vi "Run Test.vi"(8 "error in (no error)":errorcluster, 11 "Test Template in":refnum<class "Instrument Setup.lvclass">) -> (0 "error out":errorcluster, 1 "Positions":i32[](array[numeric]), 2 "Tests Passed":bool[](array[boolean]), 3 "Test Template out":refnum<class "Instrument Setup.lvclass">, 5 "Fail Codes":string[](array[string]))   [LabVIEW 2015, in "Instrument Setup.lvclass"]
doc: "Setup Loads, DPMs, Power Supplies, and Switch."
uses:
  Instrument Setup.lvclass
  CBTF Applications/Driver Board Testing/Main/Application/Application/Class/typedefs/Instrument Selector -- Enum.ctl
  Test Class/Test Class.lvclass
  CBTF Applications/Driver Board Testing/Main/Application/Application/Class/Driver Board Test.lvclass
  Classes/Application/Class/Application.lvclass
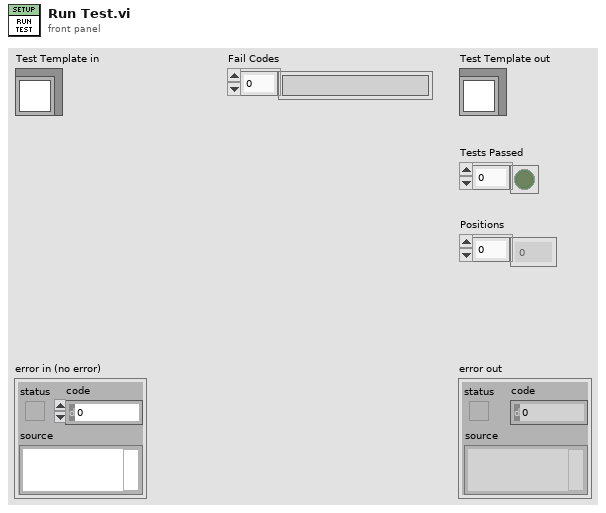
[diagram p1: front panel]
types:
  T1 = typedef "Driver Board Test.lvlib/Driver Board Test.lvclass/Instrument Selector -- Enum.ctl" = enum16{"ACPS1", "ACPS2", "DCPS1", "DCPS2", "DCPS3", "DCLoad1", "DCLoad2", "DPM1", "DPM2", "Switch1", "PXI1Slot2", "PXI1Slot3", "cDAQ1Mod5", "cDAQ1Mod6", "cDAQ1Mod7", "cDAQ1Mod8", "cDAQ1Mod1", "cDAQ1Mod2", "cDAQ1Mod3", "cDAQ1Mod4", "cDAQ2Mod1", "cDAQ2Mod2", "cDAQ2Mod3", "cDAQ2Mod4"}
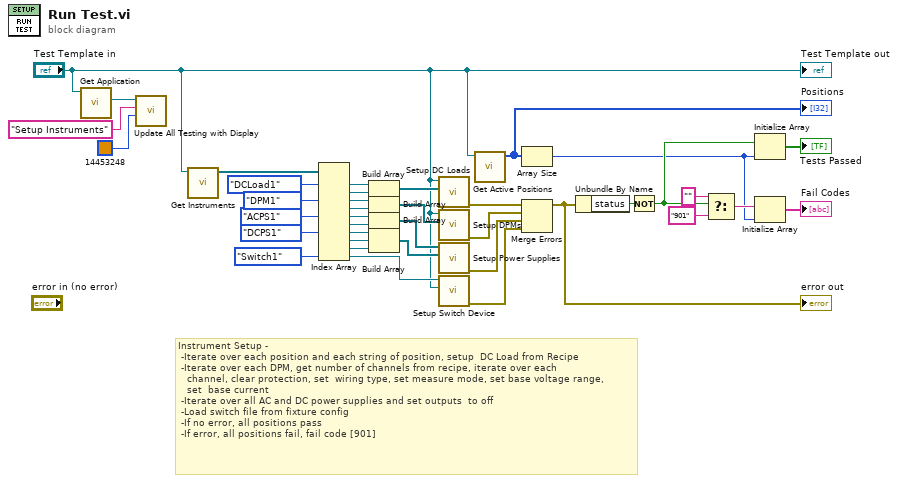
[diagram p0: block diagram]
diagram:
  # "Instrument Setup - \n\t-Iterate over each position and each string of position, setup \tDC Load from Recipe\n\t-Iterate over each DPM, get number of channels from\trecipe, iterate over each \n   channel, clear protection, set \twiring type, set measure mode, set base voltage range, \n   set \tbase current\n\t-Iterate over all AC and DC power supplies and set outputs \tto off\n\t-Load switch file from fixture config\n\t-If no error, all positions pass\n\t-If error, all positions fail, fail code [901]"
  n1 = call "Get Application.vi"("Test Class in"="Test Template in") -> ("Application.lvlib:Application.lvclass"=w7:refnum<class "Application.lvclass">)  [unwired: 9 in, 1 out]
  n2 = call "Update All Testing with Display.vi"("BG Color"=u32 14453248, "Message ('')"="Setup Instruments", "Application in"=w7) -> ()  [unwired: 7 in, 2 out]
  n3 = call "Get Instruments.vi"("Test Class in"="Test Template in") -> ("Instruments"=w5:refnum<class "Instrument.lvclass">[])  [unwired: 9 in, 1 out]
  n4 = Index Array(array=w5, index #1=Instrument_Selector_--_Enum."DCLoad1" ("Instrument"), index #3=Instrument_Selector_--_Enum."DPM1" ("Instrument"), index #5=Instrument_Selector_--_Enum."ACPS1" ("Instrument"), index #7=Instrument_Selector_--_Enum."DCPS1" ("Instrument"), index #10=Instrument_Selector_--_Enum."Switch1" ("Instrument")) -> (element #1=w18:refnum<class "Instrument.lvclass">, element #2=w17:refnum<class "Instrument.lvclass">, element #3=w20:refnum<class "Instrument.lvclass">, element #4=w19:refnum<class "Instrument.lvclass">, element #5=w25:refnum<class "Instrument.lvclass">, element #6=w24:refnum<class "Instrument.lvclass">, element #7=w23:refnum<class "Instrument.lvclass">, element #8=w22:refnum<class "Instrument.lvclass">, element #9=w21:refnum<class "Instrument.lvclass">, element #10=w8:refnum<class "Instrument.lvclass">)  [unwired: 5 in]
  n5 = Build Array(w18, w17) -> (w37:refnum<class "Instrument.lvclass">[])
  n6 = Build Array(w20, w19) -> (w28:refnum<class "Instrument.lvclass">[])
  n7 = Build Array(w25, w24) -> (w15:refnum<class "Instrument.lvclass">[])
  n8 = Build Array(w23, w22, w21) -> (w16:refnum<class "Instrument.lvclass">[])
  n9 = call "Setup DC Loads.vi"("DC Loads"=w37, "Test Class in"="Test Template in") -> ("Error out"=w36:errorcluster)  [unwired: 9 in]
  n10 = call "Setup DPMs.vi"("DPMs"=w28, "Test Class in"="Test Template in") -> ("Error out"=w27:errorcluster)  [unwired: 9 in]
  n11 = call "Setup Power Supplies.vi"("DC Supplies"=w16, "AC Supplies"=w15) -> ("error out"=w12:errorcluster)  [unwired: 9 in]
  n12 = call "Setup Switch Device.vi"("Test Class in"="Test Template in", "Instrument in"=w8) -> ("error out"=w11:errorcluster)  [unwired: 9 in]
  n13 = call "Get Active Positions.vi"("Test Class in"="Test Template in") -> ("Active Positions"=w3:u32[])  [unwired: 9 in, 1 out]
  "Positions" <- w3
  n14 = Array Size(array=w3) -> (size(s)=w31:i32)
  n15 = Merge Errors(w36, w27, w12, w11) -> (w2:errorcluster)
  "error out" <- w2
  n16 = Unbundle By Name(w2) -> ("status"=w35:bool)
  n17 = Not(x=w35) -> (.not. x?=w34:bool)
  n18 = Select(t="", s=w34, f="901") -> (s? t:f=w32:string)
  n19 = Initialize Array(w34, w31) -> (→"Tests Passed":bool[])
  n20 = Initialize Array(w32, w31) -> (→"Fail Codes":string[])
  "Test Template out" <- "Test Template in"
